vi "Write Last Voltages.vi"(8 "error in (no error)":errorcluster, 10 "Last Voltage":map{u8, dbl}(c390), 11 "Scope Base in":refnum<class "Scope Base.lvclass">) -> (0 "error out":errorcluster, 3 "Scope Base out":refnum<class "Scope Base.lvclass">)   [LabVIEW 2023, in "Scope Base.lvlib" / "Scope Base.lvclass"]
uses:
  Scope Base.lvclass
  Scope Base.lvclass/Scope Base.ctl
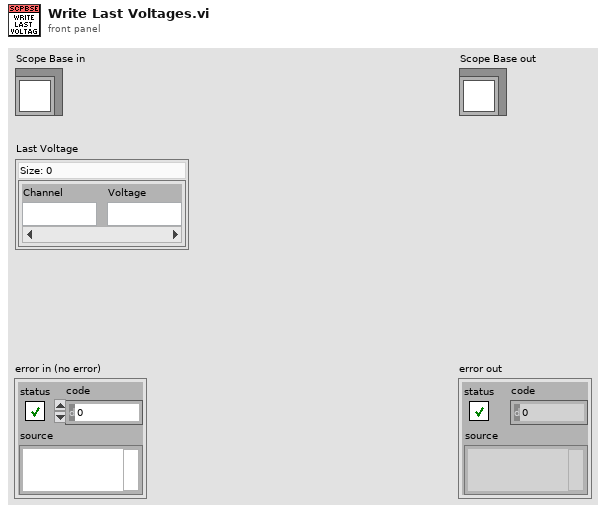
[diagram p1: front panel]
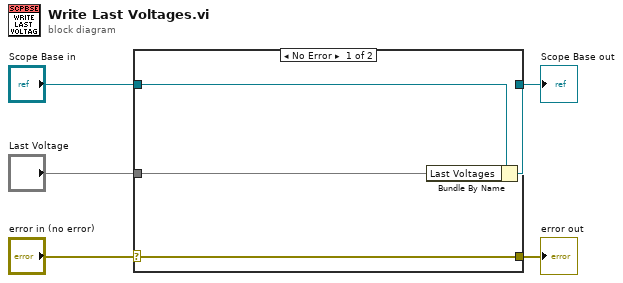
[diagram p0: block diagram]
diagram:
  n1 = case shown="No Error" "error in (no error)" {
    selector: "error in (no error)" -> [w9 w10]
    tunnel: [w9 w10] -> w4
    tunnel: [w7 w11] -> w2
    tunnel: "Scope Base in" -> [w8 w11]
    tunnel: "Last Voltage" -> [w6 _]
    frame No Error {
      n2 = Bundle By Name(cluster=w8, "Last Voltages"=w6) -> (w7:refnum<class "Scope Base.lvclass">)
    }
    frame Error {
    }
  }
  "error out" <- w4
  "Scope Base out" <- w2
